vi "Set Error (Owner).vi"(8 "error in (no error)":errorcluster, 9 "error list <owner>":variant, 10 "owner":string, 11 "error list <scope> in":variant) -> (0 "error out":errorcluster, 3 "error list <scope> out":variant)   [LabVIEW 2017]
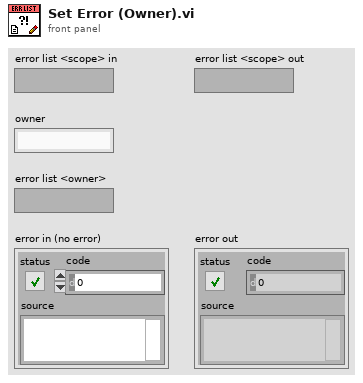
[diagram p1: front panel]
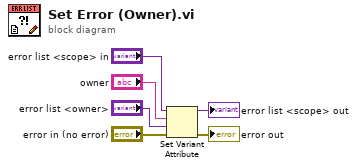
[diagram p0: block diagram]
diagram:
  n1 = Set Variant Attribute(Variant="error list <scope> in", name="owner", value="error list <owner>", error in="error in (no error)") -> (Variant out=→"error list <scope> out":variant, error out=→"error out":errorcluster)  [unwired: 1 out]
